vi "Format Result.vi"(1 "Pass?":bool[](array[boolean]), 2 "VI names":string[](array[string])) -> (0 "Result":string)   [LabVIEW 2019, in "UnitTestFramework.lvclass"]
uses:
  UnitTestFramework.lvclass
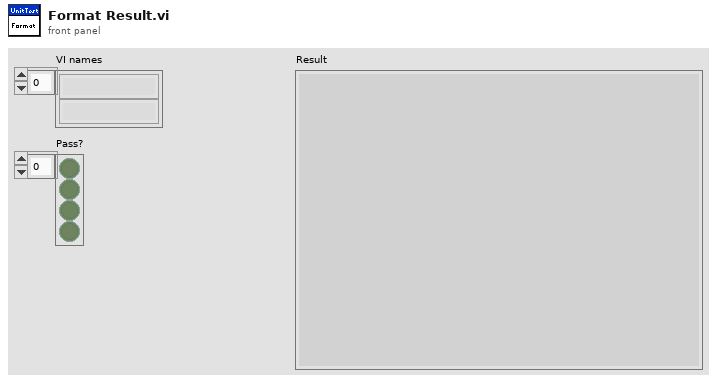
[diagram p1: front panel]
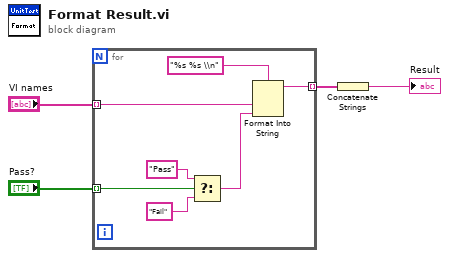
[diagram p0: block diagram]
diagram:
  n1 = for {
    tunnel: "VI names" -> [w10] mode=indexing
    tunnel: "Pass?" -> [w9] mode=indexing
    tunnel: [w5] -> w2 mode=indexing
    n2 = Select(t="Pass", s=w9, f="Fail") -> (s? t:f=w6:string)
    n3 = Format Into String(format string="%s %s \\n", w10, w6) -> (resulting string=w5:string)  [unwired: 2 in, 1 out]
  }
  n4 = Concatenate Strings(w2) -> (→"Result":string)
